vi "cdex_Position PID.vi"(10 "states":dbl[](array[numeric]) format="%.2f", 11 "travel":dbl) -> (2 "Output (u)":dbl)   [LabVIEW 2011]
uses:
  <vilib>/Simulation/Implementation/Shared/SIMSCR Execution Mode.ctl
  <vilib>/Simulation/Scripting/Companion Diagram/SimConfigNode/SimParams.ctl
  <vilib>/Simulation/Scripting/Companion Diagram/SimConfigNode/_simSolvers.ctl
  <vilib>/Simulation/Param Hierarchy/Typedefs/SIMPH Param Control Actions.ctl
  <vilib>/Simulation/Implementation/Shared/SIM limit type.ctl
  <vilib>/Simulation/SignalArithmetic/Implementation/NILVSim Gain.llb/SIM Gain (scalar).vi
  <vilib>/Simulation/Nonlinear/Implementation/NILVSim Saturation.llb/SIM Saturation (scalar).vi
  <vilib>/Simulation/ContinuousLinear/Implementation/NILVSim Integrator new.llb/SIM Integrator distributor (scalar).vi
  <vilib>/Simulation/ContinuousLinear/Implementation/NILVSim Integrator new.llb/SIM Integrator collector (scalar).vi
  <vilib>/Simulation/Implementation/Shared/NILVSim_Manager.vi
  <vilib>/Simulation/Implementation/Shared/NILVSim_ParamChanged.vi
  <vilib>/Simulation/Implementation/Shared/NILVSim_FinalizeModel.vi
  <vilib>/Simulation/Implementation/Shared/SIM Unbundle Sim Info.vi
  <vilib>/Simulation/Implementation/Shared/NILVSim_GetModelError.vi
  <vilib>/Simulation/Implementation/Shared/SIM SimErrorHandler.vi
  <vilib>/Simulation/Implementation/Shared/SIM Bundle Sim Info.vi
  3DHe_Global.vi
  <vilib>/Simulation/Implementation/Shared/NILVSim_Initialize.vi
  <vilib>/Simulation/Scripting/Companion Diagram/SimConfigNode/SimDog.xnode
  <vilib>/Simulation/Implementation/XNodeFramework/SimXNode/SimX.xnode
  <vilib>/Simulation/ContinuousLinear/Implementation/NILVSim Integrator new.llb/SIM Integrator (scalar).vi
  <vilib>/Simulation/Implementation/Shared/NI_SIM_Implementation.lvlib
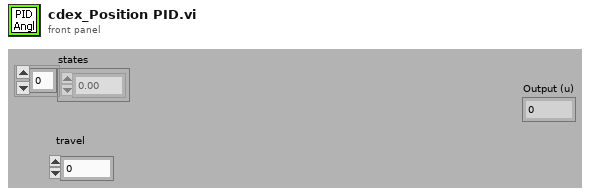
[diagram p1: front panel]
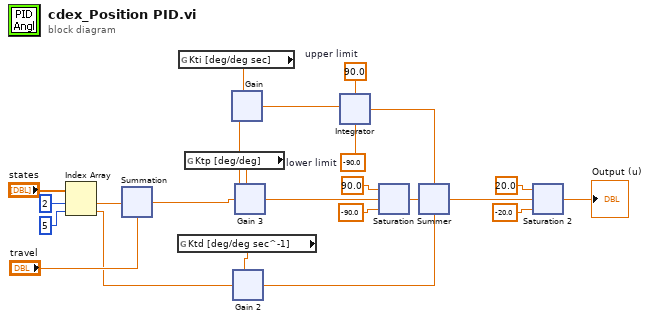
[diagram p0: block diagram]
diagram:
  w13 = -90.0  # lower limit
  w14 = 90.0  # upper limit
  n1 = Index Array(array="states", index #1=2 ("index"), index #2=5 ("index")) -> (element #1=w18:dbl, element #2=w15:dbl)
  n2 = xnode ("Summation")("Operand1"=w18, "Operand2"="travel") -> ("Result"=w1:dbl)
  n3 = global read "3DHe_Global.vi" "Ktd [deg/deg sec^-1]"() -> (w2:dbl)
  n4 = global read "3DHe_Global.vi 2" "Kti [deg/deg sec]"() -> (w3:dbl)
  n5 = global read "3DHe_Global.vi 3" "Ktp [deg/deg]"() -> (w4:dbl)
  n6 = xnode ("Gain")("gain"=w3, "input"=w1) -> ("output"=w23:dbl)  [unwired: 2 in]
  n7 = xnode ("Gain 2")("gain"=w2, "input"=w15) -> ("output"=w16:dbl)  [unwired: 2 in]
  n8 = xnode ("Gain 3")("gain"=w4, "input"=w1) -> ("output"=w5:dbl)  [unwired: 2 in]
  n9 = xnode ("Integrator")("upper limit"=w14, "input"=w23, "lower limit"=w13) -> ("output"=w22:dbl)  [unwired: 7 in, 2 out]
  n10 = xnode ("Saturation")("upper limit"=90.0, "input"=w5, "lower limit"=-90.0) -> ("output"=w6:dbl)  [unwired: 2 in]
  n11 = xnode ("Summer")("Operand1"=w22, "Operand2"=w6, "Operand3"=w16) -> ("Result"=w9:dbl)
  n12 = xnode ("Saturation 2")("upper limit"=20.0, "input"=w9, "lower limit"=-20.0) -> ("output"=→"Output (u)":dbl)  [unwired: 2 in]
